vi "Data Type to U32 1D.vi"(8 "error in (no error)":errorcluster, 11 "Data Type":refnum<class "Data Type.lvclass">) -> (0 "error out":errorcluster, 3 "U32 1D out":u32[](array[numeric]))   [LabVIEW 2017, in "U32 1D.lvclass"]
uses:
  <vilib>/gpm_packages/@cs/data-type-serializer/source/U32 1D/U32 1D.lvclass
  <vilib>/gpm_packages/@cs/data-type-serializer/source/Data Type/Data Type.lvclass
  <vilib>/gpm_packages/@cs/data-type-serializer/source/U32 1D/U32 1D.lvclass/U32 1D.ctl
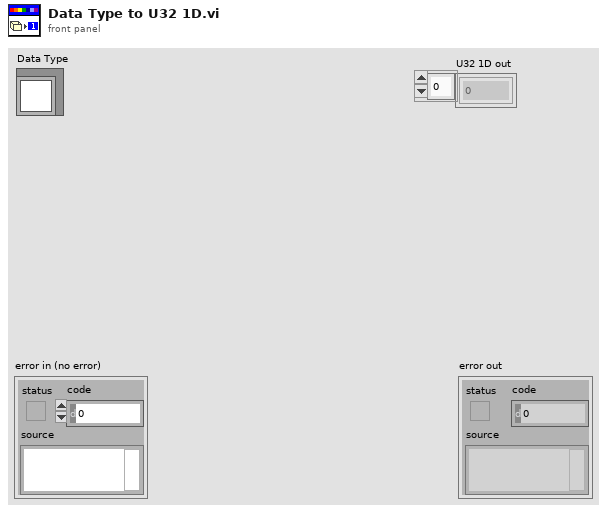
[diagram p1: front panel]
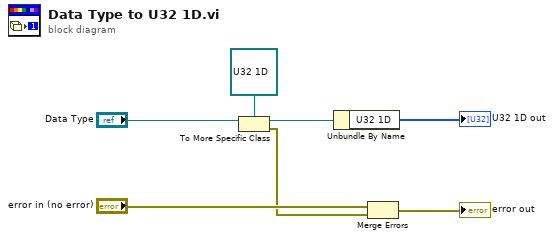
[diagram p0: block diagram]
diagram:
  n1 = To More Specific Class(target class=refnum<class "U32 1D.lvclass"> refnum ("Boolean out"), reference="Data Type") -> (specific class reference=w4:refnum<class "U32 1D.lvclass">, error out=w2:errorcluster)  [unwired: 1 in]
  n2 = Unbundle By Name(w4) -> ("U32 1D"=→"U32 1D out":u32[])
  n3 = Merge Errors("error in (no error)", w2) -> (→"error out":errorcluster)
